vi "AN97005H-Read.vi"(8 "error in":errorcluster caption="错误输入（无错误）", 11 "MyIndex":u8) -> (0 "error out":errorcluster caption="错误输出", 1 "频率":dbl, 2 "电流":dbl, 3 "电压":dbl, 5 "功率(0.1W)":dbl)   [LabVIEW 2015, in "AN97005N.lvlib"]
uses:
  AN97005N.lvlib
  <vilib>/Instr/_visa.llb/VISA Configure Serial Port (Instr).vi
panel:
  out "buff":string
  out "AC电源":refnum<visa-resource-name>
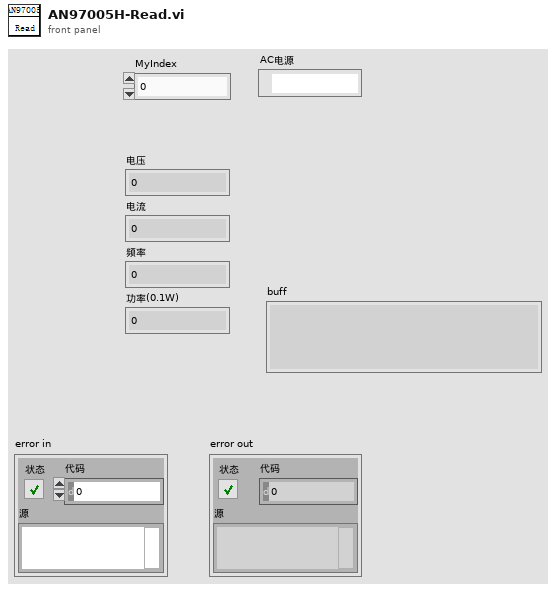
[diagram p1: front panel]
types:
  T1 = cluster{"[0]":dbl, "[1]":dbl, "[2]":dbl, "[3]":dbl}
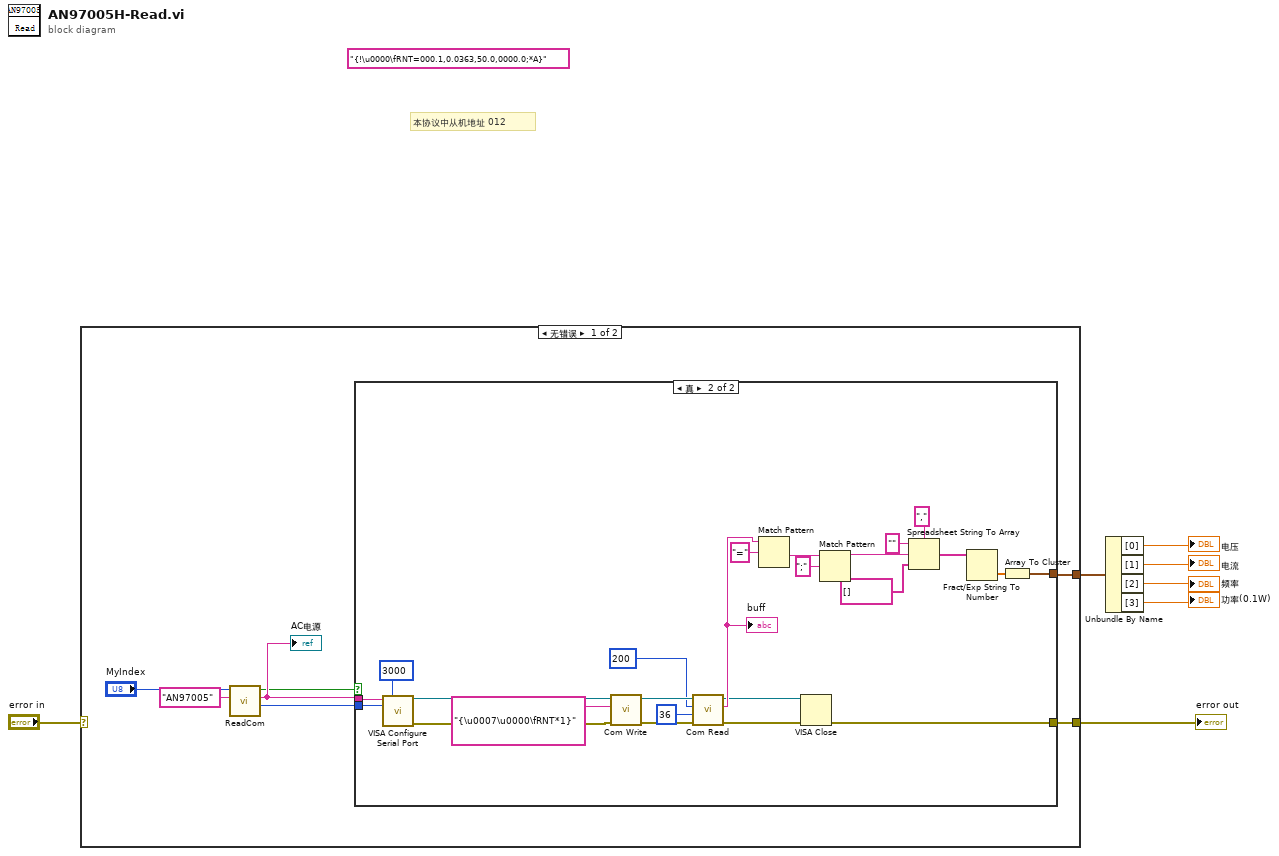
[diagram p0: block diagram]
diagram:
  (unwired) "{!\u0000\fRNT=000.1,0.0363,50.0,0000.0;*A}"
  # "本协议中从机地址 012"
  n1 = case shown="无错误" "error in" {
    selector: "error in" -> [_ w39]
    tunnel: [w9 _] -> w7
    tunnel: [w8 w39] -> w2
    frame No Error {
      n2 = call "ReadCom.vi"("仪器名称"="AN97005", "MyIndex"="MyIndex") -> ("Baudrate"=w10:i32, "COM"=w12:string, "OK?"=w11:bool)  [unwired: 7 in]
      "AC电源" <- w12
      n3 = case shown="真" w11 {
        tunnel: [_ w21] -> w9
        tunnel: w12 -> [_ w20]
        tunnel: w10 -> [_ w16]
        tunnel: [_ w15] -> w8
        frame False {
        }
        frame True {
          n4 = call-poly "VISA Configure Serial Port"("VISA resource name"=w20, "timeout (10sec)"=u32 3000, "baud rate (9600)"=w16) -> ("VISA resource name out"=w37:refnum<visa-resource-name>, "error out"=w19:errorcluster)  [unwired: 11 in]
          n5 = call "Com Write.vi"("错误输入（无错误）"=w19, "Wbuff"="{\u0007\u0000\fRNT*1}", "VISA In"=w37) -> ("错误输出"=w34:errorcluster, "VISA Out"=w35:refnum<visa-resource-name>)  [unwired: 7 in]
          n6 = call "Com Read.vi"("错误输入（无错误）"=w34, "num"=u32 36, "超时"=u32 200, "VISA In"=w35) -> ("错误输出"=w38:errorcluster, "buff"=w23:string, "VISA Out"=w18:refnum<visa-resource-name>)  [unwired: 5 in]
          "buff" <- w23
          n7 = Match Pattern(string=w23, regular expression="=" ("正则表达式")) -> (after substring=w30:string)  [unwired: 1 in, 3 out]
          n8 = VISA Close(VISA resource name=w18, error in (no error)=w38) -> (error out=w15:errorcluster)
          n9 = Match Pattern(string=w30, regular expression=";" ("正则表达式")) -> (before substring=w27:string)  [unwired: 1 in, 3 out]
          n10 = Spreadsheet String To Array(delimiter (Tab)="," ("分隔符(Tab)"), format string="" ("格式字符串"), spreadsheet string=w27, array type (2D Dbl)=string[] []) -> (array=w24:string[])
          n11 = Fract/Exp String To Number(string=w24) -> (number=w22:dbl[])  [unwired: 3 in, 1 out]
          n12 = Array To Cluster(array=w22) -> (cluster=w21:T1)
        }
      }
    }
    frame Error {
    }
  }
  "error out" <- w2
  n13 = Unbundle By Name(w7) -> ("[0]"=→"电压":dbl, "[1]"=→"电流":dbl, "[2]"=→"频率":dbl, "[3]"=→"功率(0.1W)":dbl)
